vi "Sort_event_array.vi"(11 "Data cluster in":T1) -> (0 "sorted event array":string[](array[string]))   [LabVIEW 2017, in "labview-standard-library.lvlib" / "data-logging.lvlib"]
doc: "Sorts the events based on which happened first in case the asynchronous nature of the queueing system causes events to be written out of order."
uses:
  data-logging.lvlib
  Event_log_binary_data.ctl
  Time&Event_cluster.ctl
panel:
  # "Sorts the events based on which happened first in case the asynchronous nature of the queueing system causes events to be written out of order, with respect to time."
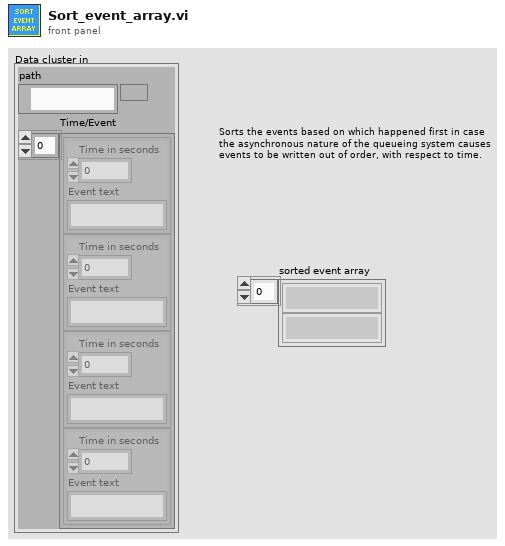
[diagram p1: front panel]
types:
  T1 = typedef "labview-standard-library.lvlib/data-logging.lvlib/Event_log_binary_data.ctl" = cluster{"path":path, "Time/Event":T2[]}
  T2 = typedef "labview-standard-library.lvlib/data-logging.lvlib/Time&Event_cluster.ctl" = cluster{"Time in seconds":dbl, "Event text":string}
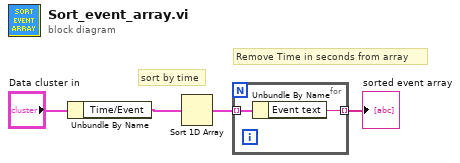
[diagram p0: block diagram]
diagram:
  # "Remove Time in seconds from array"
  # "sort by time"
  n1 = Unbundle By Name("Data cluster in") -> ("Time/Event"=w3:T2[])
  n2 = Sort 1D Array(array=w3) -> (sorted array=w1:T2[])
  n3 = for {
    tunnel: w1 -> [w6] mode=indexing
    tunnel: [w5] -> w2 mode=indexing
    n4 = Unbundle By Name(w6) -> ("Event text"=w5:string)
  }
  "sorted event array" <- w2
